vi "receive.vi"(8 "error in (no error)":errorcluster, 11 "Redis Pipelining TCP Client in":refnum<class "Redis Pipelining TCP Client.lvclass">) -> (0 "error out":errorcluster, 1 "timed out?":bool, 2 "RESP3 Value":variant, 3 "Redis Pipelining TCP Client out":refnum<class "Redis Pipelining TCP Client.lvclass">)   [LabVIEW 2019, in "Redis Client for LabVIEW.lvlib" / "Redis Pipelining TCP Client.lvclass"]
uses:
  Redis Pipelining TCP Client.lvclass
  Redis Pipelining TCP Client.lvclass/Redis Pipelining TCP Client.ctl
  Redis TCP Client/Redis TCP Client.lvclass
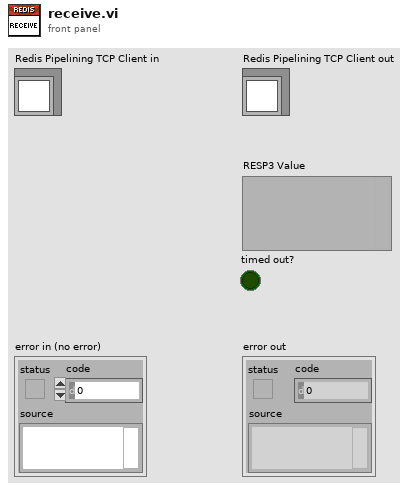
[diagram p1: front panel]
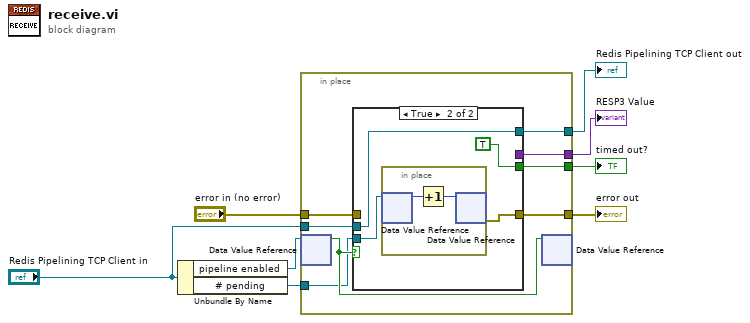
[diagram p0: block diagram]
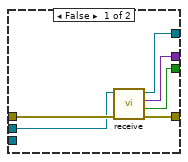
[diagram p2: hidden frame]
diagram:
  n1 = Unbundle By Name("Redis Pipelining TCP Client in") -> ("pipeline enabled"=w2:refnum<data-value>, "# pending"=w1:refnum<data-value>)
  n2 = in-place {
    in-place-border: "error in (no error)" -> [w15]
    in-place-border: "Redis Pipelining TCP Client in" -> [w14]
    in-place-border: w1 -> [w13]
    in-place-border: [w12] -> w3
    in-place-border: [w11] -> w8
    in-place-border: [w10] -> w7
    in-place-border: [w9] -> w5
    n3 = in-place-dvr #1(w2) -> (w16:bool)  [unwired: 1 out]
    n4 = case shown="True" w16 {
      tunnel: [w22 w23] -> w12
      tunnel: [w21 TRUE ("timed out?")] -> w11
      tunnel: [w20 _] -> w10
      tunnel: [w19 w26] -> w9
      tunnel: w15 -> [w18 _]
      tunnel: w14 -> [w17 w26]
      tunnel: w13 -> [_ w24]
      frame False {
        n5 = call-parent "receive.vi"("error in (no error)"=w18, "Redis TCP Client in"=w17) -> ("error out"=w22:errorcluster, "timed out?"=w21:bool, "RESP3 Value"=w20:variant, "Redis TCP Client out"=w19:refnum<class "Redis Pipelining TCP Client.lvclass">)  [unwired: 6 in]
      }
      frame True {
        n6 = in-place {
          n7 = in-place-dvr #2(w24) -> (w28:i32)  [unwired: 1 out]
          n8 = Increment(x=w28) -> (x+1=w27:i32)
          n9 = in-place-dvr #2(w27) -> (w23:errorcluster)  [unwired: 1 out]
        }
      }
    }
    n10 = in-place-dvr #1(w16) -> ()  [unwired: 2 out]
  }
  "error out" <- w3
  "Redis Pipelining TCP Client out" <- w5
  "RESP3 Value" <- w7
  "timed out?" <- w8
